vi "Get Optimisation Status.vi"(8 "error in (no error)":errorcluster, 11 "Run Block in":refnum<class "Run Block.lvclass">) -> (0 "error out":errorcluster, 2 "Optimiser":bool, 3 "Run Block out":refnum<class "Run Block.lvclass">)   [LabVIEW 2020, in "TALOS.lvlib" / "Run Utilities.lvlib" / "Run Block.lvclass"]
doc: "VI checks if the next active cell is an optimisation cell"
uses:
  Run Block.lvclass
  Run Block.lvclass/Run Block.ctl
  Schedule/Schedule.lvclass
  Cell/Schedule Cell.lvclass
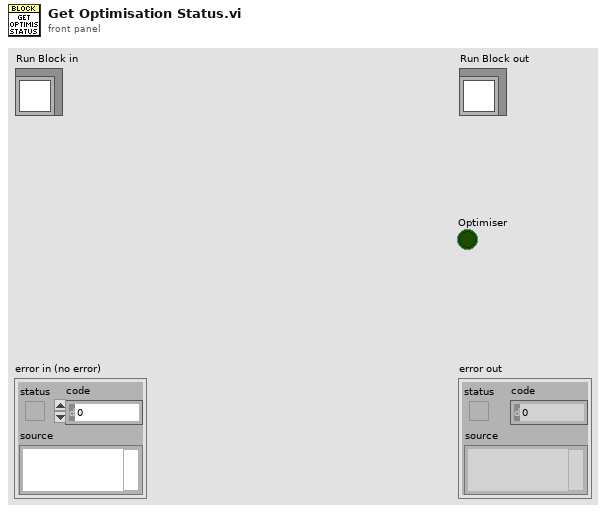
[diagram p1: front panel]
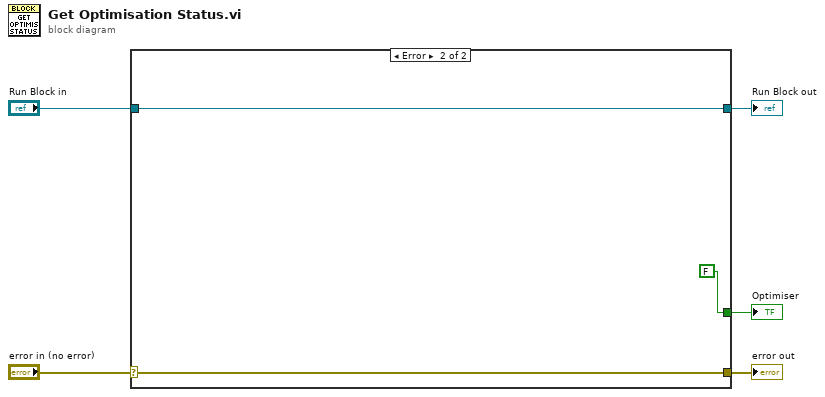
[diagram p0: block diagram]
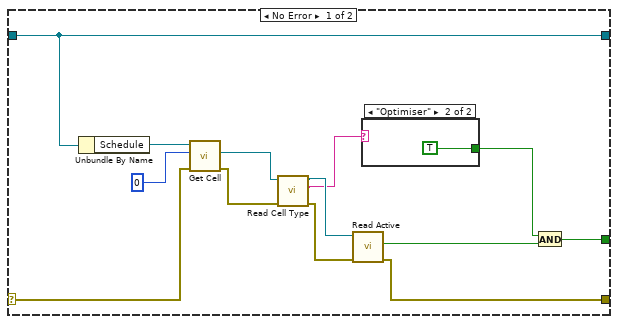
[diagram p2: hidden frame]
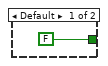
[diagram p3: hidden frame]
diagram:
  n1 = case shown="Error" "error in (no error)" {
    selector: "error in (no error)" -> [w16 w23]
    tunnel: [w11 w23] -> w4
    tunnel: [w18 w22] -> w2
    tunnel: "Run Block in" -> [w18 w22]
    tunnel: [w12 FALSE ("Optimiser")] -> w1
    frame No Error {
      n2 = Unbundle By Name(w18) -> ("Schedule"=w17:refnum<class "Schedule.lvclass">)
      n3 = call-dynamic "Get Cell.vi"("error in (no error)"=w16, "index"=0, "Schedule in"=w17) -> ("error out"=w6:errorcluster, "Schedule Cell"=w10:refnum<class "Schedule Cell.lvclass">)  [unwired: 6 in, 1 out]
      n4 = call-dynamic "Read Cell Type.vi"("error in (no error)"=w6, "Schedule Cell in"=w10) -> ("error out"=w7:errorcluster, "Cell Type"=w8:string, "Schedule Cell out"=w9:refnum<class "Schedule Cell.lvclass">)  [unwired: 7 in]
      n5 = call-dynamic "Read Active.vi"("error in (no error)"=w7, "Schedule Cell in"=w9) -> ("error out"=w11:errorcluster, "Active"=w14:bool)  [unwired: 7 in, 1 out]
      n6 = case shown="\"Optimiser\"" w8 {
        tunnel: [FALSE ("Optimiser") TRUE ("Optimiser")] -> w13
        frame Default {
        }
        frame "Optimiser" {
        }
      }
      n7 = And(x=w13, y=w14) -> (x .and. y?=w12:bool)
    }
    frame Error {
    }
  }
  "error out" <- w4
  "Run Block out" <- w2
  "Optimiser" <- w1
